vi "stream_data.vi"(7 "timeout in ms (-1)":i32, 8 "error in (no error)":errorcluster, 9 "Display":refnum<notifier>, 10 "Response":refnum<notifier>, 11 "Command":refnum<notifier>) -> (0 "error out":errorcluster)   [LabVIEW 2018]
uses:
  controls/Sensor_Data.ctl
  controls/MAG_UI_Command.ctl
  controls/MAG_Comms_State.ctl
panel:
  out "timed out?":bool
  out "response":string
  in  "Update Delay (dT)":i32(slide)=100 scale=20.0..100.0
  out "Streaming Data IO":bool
  in  "Stop Button":bool
  out "dT":i32
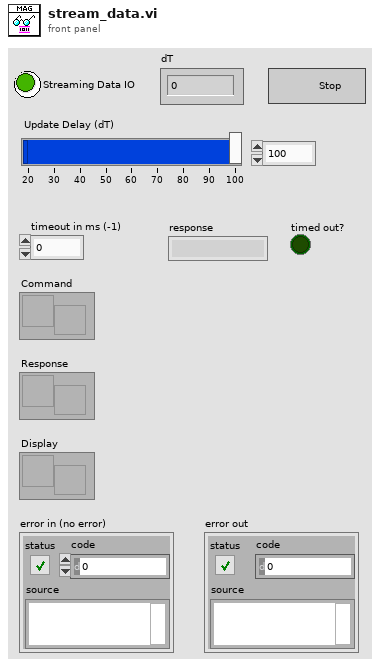
[diagram p1: front panel]
types:
  T1 = typedef "Sensor_Data.ctl" = cluster{"Time":u32, "Data":i16[]}
  T2 = typedef "MAG_UI_Command.ctl" = cluster{"Comms_States":T3, "Parameters":string, "Clear Buffer?":bool}
  T3 = typedef "MAG_Comms_State.ctl" = enum16{"Initialize", "Wait for Event", "Connect", "Send_Com", "Rcv_TXT", "Rcv_BIN", "Rcv_FILE", "Disconnect"}
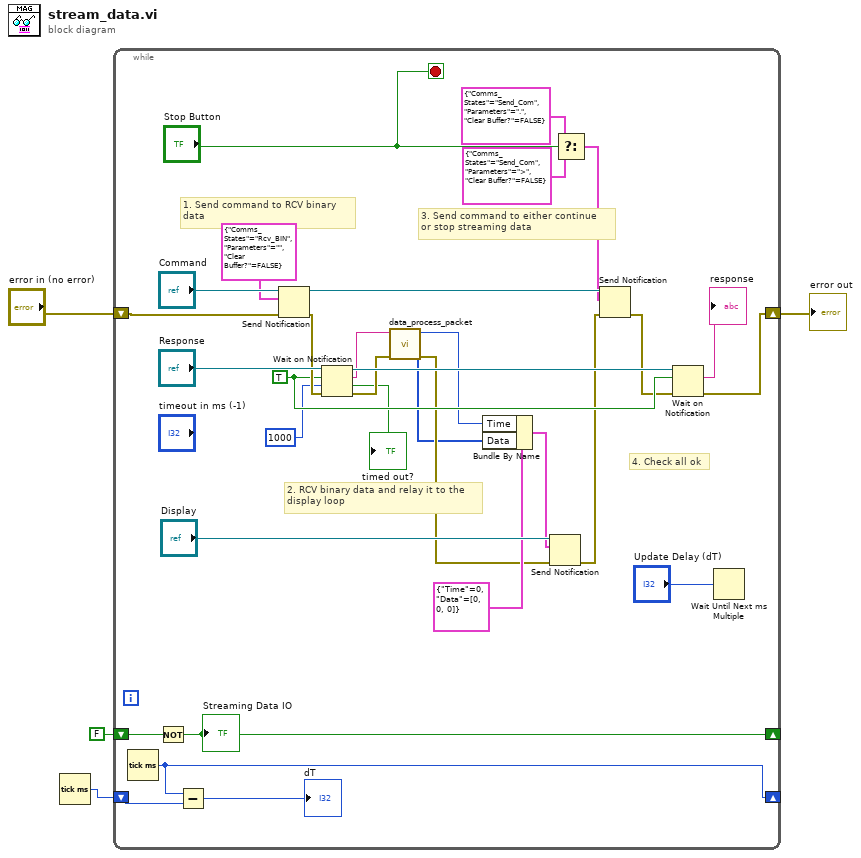
[diagram p0: block diagram]
diagram:
  n1 = Tick Count (ms)() -> (millisecond timer value=w1:u32)
  n2 = while {
    shift-right: [w21] -> w3
    shift-left: "error in (no error)" -> [w22]
    shift-right: [w18] -> _
    shift-left: FALSE -> [w19]
    shift-right: [w8] -> _
    shift-left: w1 -> [w10]
    stop <- "Stop Button" stop-if-true
    w26 = TRUE ("ignore previous (F)")
    # "4. Check all ok"
    # "3. Send command to either continue\nor stop streaming data"
    # "2. RCV binary data and relay it to the \ndisplay loop"
    # "1. Send command to RCV binary\ndata"
    n3 = Tick Count (ms)() -> (millisecond timer value=w8:u32)
    n4 = Not(x=w19) -> (.not. x?=w18:bool)
    "Streaming Data IO" <- w18
    n5 = Subtract(x=w8, y=w10) -> (x-y=→"dT":u32)
    n6 = Send Notification(notification=T2 {"Comms_States"=enum."Rcv_BIN", "Parameters"="", "Clear Buffer?"=FALSE}, notifier="Command", error in (no error)=w22) -> (notifier out=w31:refnum<notifier>, error out=w34:errorcluster)
    n7 = Wait on Notification(notifier="Response", ignore previous (F)=w26, timeout in ms (-1)=1000, error in (no error)=w34) -> (notifier out=w27:refnum<notifier>, notification=w17:string, timed out?=→"timed out?":bool, error out=w16:errorcluster)
    n8 = call "data_process_packet.vi"("error in (no error)"=w16, "Binary Input Data"=w17) -> ("error out"=w15:errorcluster, "Raw Sensors (Flattened)"=w12:i16[], "Time"=w14:u32)  [unwired: 5 in, 2 out]
    n9 = Bundle By Name(cluster=T1 {"Time"=0, "Data"=[0, 0, 0]} ("notification"), "Time"=w14, "Data"=w12) -> (w11:T1)
    n10 = Send Notification(notification=w11, notifier="Display", error in (no error)=w15) -> (error out=w25:errorcluster)  [unwired: 1 out]
    n11 = Select(t=T2 {"Comms_States"=enum."Send_Com", "Parameters"=".", "Clear Buffer?"=FALSE}, s="Stop Button", f=T2 {"Comms_States"=enum."Send_Com", "Parameters"=">", "Clear Buffer?"=FALSE}) -> (s? t:f=w28:T2)
    n12 = Send Notification(notification=w28, notifier=w31, error in (no error)=w25) -> (error out=w24:errorcluster)  [unwired: 1 out]
    n13 = Wait on Notification(notifier=w27, ignore previous (F)=w26, error in (no error)=w24) -> (notification=→"response":string, error out=w21:errorcluster)  [unwired: 1 in, 2 out]
    n14 = Wait Until Next ms Multiple(millisecond multiple="Update Delay (dT)") -> ()  [unwired: 1 out]
  }
  "error out" <- w3
